vi "mod_2pi.vi"(11 "state k+1":T1) -> (3 "state_mod2pi":T1)   [LabVIEW 2019]
uses:
  coordinate.ctl
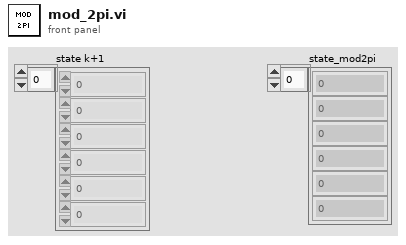
[diagram p1: front panel]
types:
  T1 = typedef "coordinate.ctl" = dbl[]
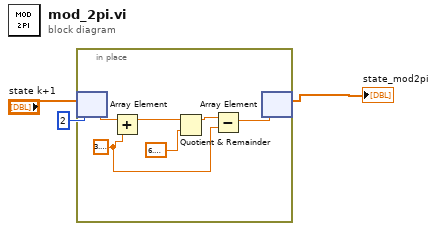
[diagram p0: block diagram]
diagram:
  n1 = in-place {
    w4 = 3.141592653589793
    n2 = in-place-array #1("state k+1", 2) -> (w9:dbl)
    n3 = Add(x=w9, y=w4) -> (x+y=w6:dbl)
    n4 = Quotient & Remainder(x=w6, y=6.283185307179586) -> (x-y*floor(x/y)=w7:dbl)  [unwired: 1 out]
    n5 = Subtract(x=w7, y=w4) -> (x-y=w5:dbl)
    n6 = in-place-array #1(w5) -> (→"state_mod2pi":T1)  [unwired: 1 out]
  }
